vi "Process Data.vi"(7 "AdasLvTemplate in":refnum<class "AdasLvTemplate.lvclass">, 8 "error in":errorcluster, 11 "Node in":refnum<class "BLS Cycler Template.lvclass">) -> (0 "error out":errorcluster, 3 "Node out":refnum<class "BLS Cycler Template.lvclass">, 5 "AdasLvTemplate out":refnum<class "AdasLvTemplate.lvclass">)   [LabVIEW 2023, in "BLS Cycler Template.lvlib" / "BLS Cycler Template.lvclass"]
uses:
  BLS Cycler Template.lvclass
  <vilib>/ADAS Replay HIL/ADAS Plugin Utilities/AdasLvTemplate/AdasLvTemplate.lvclass
  BLS Cycler Template.lvclass/BLS Cycler Template.ctl
  <vilib>/ADAS Replay HIL/ADAS Plugin Utilities/AdasLvTemplate/Typedefs/Out Of Band/Status Custom DBL Selector.ctl
  <vilib>/ADAS Replay HIL/ADAS Plugin Utilities/AdasLvTemplate/AdasLvTemplate.lvclass/AdasLvTemplate.ctl
  de41bea3-f2c7-4911-b816-388d7dc5d8a5.vi
  de41bea3-f2c7-4911-b816-388d7dc5d8a5.vi/4bc1c15b-36ab-481f-b8dd-c64075ce723a.vi
  de41bea3-f2c7-4911-b816-388d7dc5d8a5.vi/d83cb72b-7713-41fc-a3d1-682de79cf574.vi
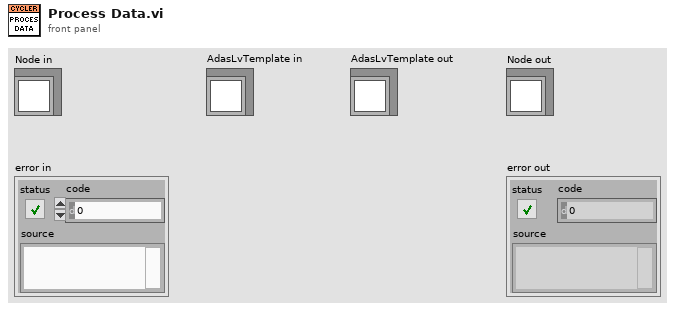
[diagram p1: front panel]
types:
  T1 = typedef "AdasLvTemplate.lvlib/AdasLvTemplate.lvclass/Status Custom DBL Selector.ctl" = enum16{"Custom 5 (DBL)", "Custom 6 (DBL)", "Custom 7 (DBL)", "Custom 8 (DBL)"}
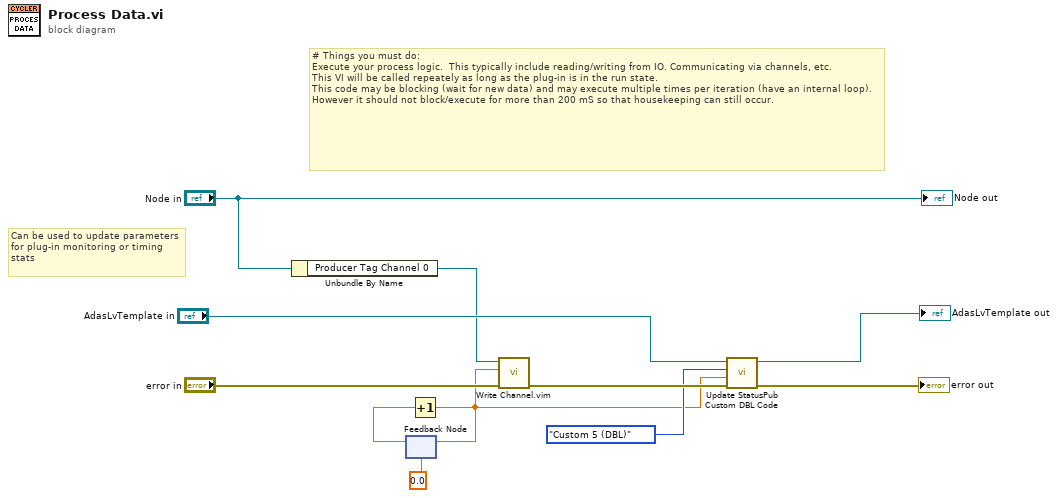
[diagram p0: block diagram]
diagram:
  # "# Things you must do:\nExecute your process logic.  This typically include reading/writing from IO. Communicating via channels, etc.  \nThis VI will be called repeately as long as the plug-in is in the run state.\nThis code may be blocking (wait for new data) and may execute multiple times per iteration (have an internal loop).  However it should not block/execute for more than 200 mS so that housekeeping can still occur."
  # "Can be used to update parameters for plug-in monitoring or timing stats"
  n1 = Unbundle By Name("Node in") -> ("Producer Tag Channel 0"=w3:refnum<k21>)
  n2 = feedback #1(0.0) -> (w9:dbl)
  n3 = Increment(x=w9) -> (x+1=w2:dbl)
  n4 = feedback-in #1(w2) -> ()
  n5 = call "Write Channel.vim"("error in"="error in", "Data in"=w2, "ADAS HIL Channel in"=w3) -> ("error out"=w11:errorcluster)  [unwired: 6 in, 2 out]
  n6 = call <vilib>:"Update StatusPub Custom DBL Code.vi"("error in (no error)"=w11, "Custom Data"=w2, "Terminal"=Status_Custom_DBL_Selector."Custom 5 (DBL)", "AdasLvTemplate in"="AdasLvTemplate in") -> ("error out"=→"error out":errorcluster, "AdasLvTemplate out"=→"AdasLvTemplate out":refnum<class "AdasLvTemplate.lvclass">)  [unwired: 6 in]
  "Node out" <- "Node in"
